vi "RECEBE NOME-CLIENTE.vi"() -> ()   [LabVIEW 2019]
panel:
  out "error out":errorcluster
  in  "size":i32
  in  "stop":bool
  out "NOMES":string[](array[string])
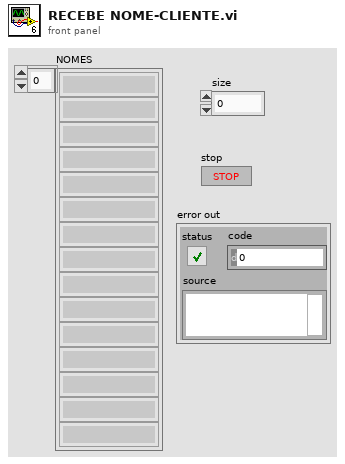
[diagram p1: front panel]
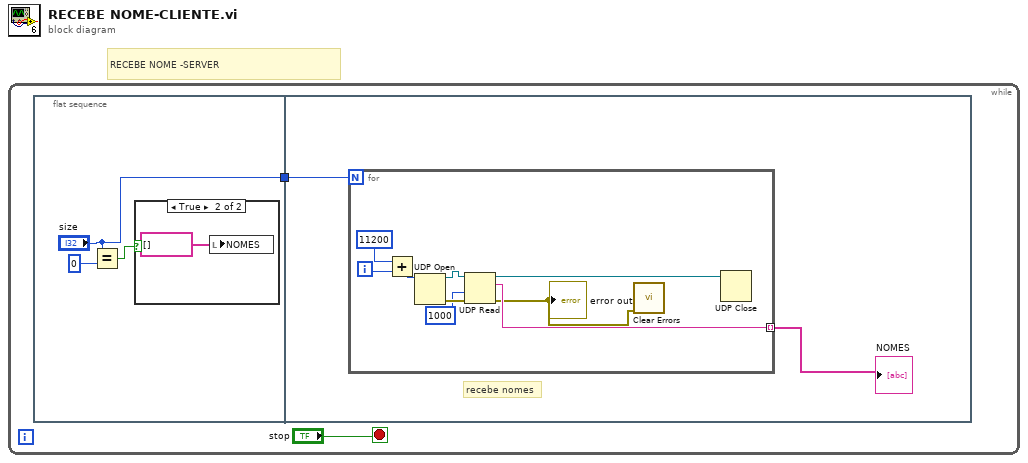
[diagram p0: block diagram]
diagram:
  # "RECEBE NOME -SERVER"
  n1 = while {
    stop <- "stop" stop-if-true
    n2 = flat-sequence {
      tunnel: ["size"] -> w1
      tunnel: w1 -> [w7]
      frame #0 {
        n3 = Equal?(x="size", y=0) -> (x = y?=w4:bool)
        n4 = case shown="True" w4 {
          frame False {
          }
          frame True {
            n5 = local write "NOMES"(string[] [] ("NOMES")) -> ()
          }
        }
      }
      frame #1 {
        # "recebe nomes"
        n6 = for {
          N: w7 -> [_]
          tunnel: [w10] -> w8 mode=indexing
          i -> [w16]
          n7 = Add(x=u16 11200 ("port"), y=w16) -> (x+y=w15:i32)
          n8 = UDP Open(11:w15) -> (port=w14:refnum<k16>, 0:w12:errorcluster)  [unwired: 4 in, 1 out]
          n9 = UDP Read(connection ID=w14, timeout ms (25000)=1000, 8:w12) -> (data out=w10:string, error out=w9:errorcluster, 3:w13:refnum<k16>)  [unwired: 1 in, 2 out]
          "error out" <- w9
          n10 = call <vilib>:"Clear Errors.vi"("error in (no error)"=w9) -> ()  [unwired: 5 in, 2 out]
          n11 = UDP Close(connection ID=w13) -> ()  [unwired: 1 in, 2 out]
        }
        "NOMES" <- w8
      }
    }
  }
